vi "YKWT230 Config Wiring.vi"(0 "VISA resource name":refnum<visa-resource-name>, 5 "Wiring (1: 1P3W)":u16(ring)=1 items=["", "1P3W", "3P3W", "3P4W", "3V3A"], 11 "error in (no error)":errorcluster) -> (4 "VISA resource name out":refnum<visa-resource-name>, 15 "error out":errorcluster)   [LabVIEW 2016, in "Yokogawa WT200 Series.lvlib"]
doc: "This VI sends the wiring method command to the WT230."
uses:
  Yokogawa WT200 Series.lvlib
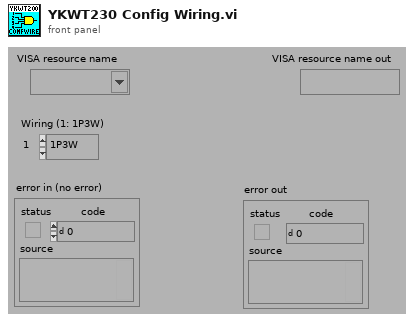
[diagram p1: front panel]
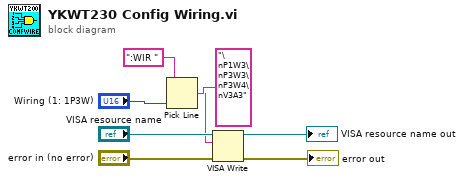
[diagram p0: block diagram]
diagram:
  n1 = Pick Line(string ("")=":WIR ", multi-line string="\nP1W3\nP3W3\nP3W4\nV3A3", line index="Wiring (1: 1P3W)") -> (output string=w1:string)
  n2 = VISA Write(VISA resource name="VISA resource name", write buffer=w1, error in (no error)="error in (no error)") -> (VISA resource name out=→"VISA resource name out":refnum<visa-resource-name>, error out=→"error out":errorcluster)  [unwired: 1 out]
